vi "Cluster to JSON.vi"(8 "error in":errorcluster, 11 "Mouse Data":T2) -> (0 "error out":errorcluster, 3 "JSON":string)   [LabVIEW 2011]
uses:
  <vilib>/Utility/GetType.llb/Type Enum.ctl
  Mouse Data Cluster.ctl
  <vilib>/vision/Image Controls.llb/IMAQ Image.ctl
  Downloads/JSON.lvlib
  <vilib>/Utility/VariantDataType/VariantType.lvlib
panel:
  out "Array":T1[](array[typedef])
  out "Type Enum":T1=enum."String"
  out "Numeric":i32
  out "Label.Text":string
  out "value":string
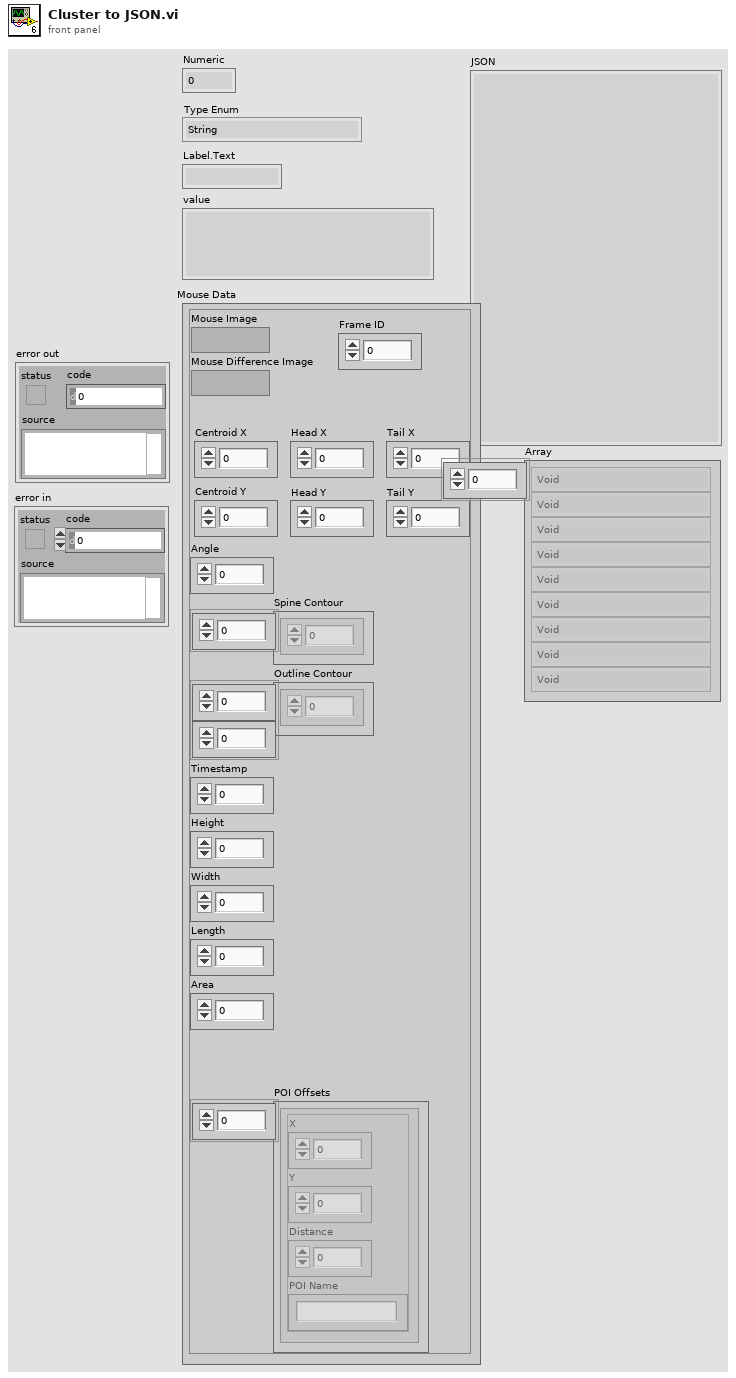
[diagram p1: front panel]
types:
  T1 = typedef "Type Enum.ctl" = enum8{"Void", "I8", "I16", "I32", "I64", "U8", "U16", "U32", "U64", "Single Float", "Double Float", "Extended Float", "Single Complex", "Double Complex", "Extended Complex", "Enum I8 NEVER", "Enum I16 NEVER", "Enum I32 NEVER", "Enum I64 NEVER", "Enum U8", "Enum U16", "Enum U32", "Enum U64", "Single Float With Unit", "Double Float With Unit", "Extended Float With Unit", "Single Complex With Unit", "Double Complex With Unit", "Extended Complex With Unit", "boolU16", "Boolean", "String", "Handle", "Path", "Picture", "C String", "Pascal String", "Tag", "SubString", "Array", "SubArray", "Cluster", "Numeric Cluster", "Variant", "LV Variant", "Measure Data (waveform)", "Refnum", "ExtData", "function", "Typedef", "Poly VI", "bad wire", "LabVIEW Class Instance"}
  T2 = typedef "Mouse Data Cluster.ctl" = cluster{"Mouse Image":T3, "Mouse Difference Image":T3, "Angle":i32, "Spine Contour":i32[], "Outline Contour":i32[][], "Timestamp":dbl, "Height":i32, "Width":i32, "Length":i32, "Area":sgl, "POI Offsets":cluster{"X":i32, "Y":i32, "Distance":i32, "POI Name":string}[], "Frame ID":i16, "Centroid X":i32, "Centroid Y":i32, "Head X":i32, "Head Y":i32, "Tail X":i32, "Tail Y":i32}
  T3 = typedef "IMAQ Image.ctl" = refnum<image>
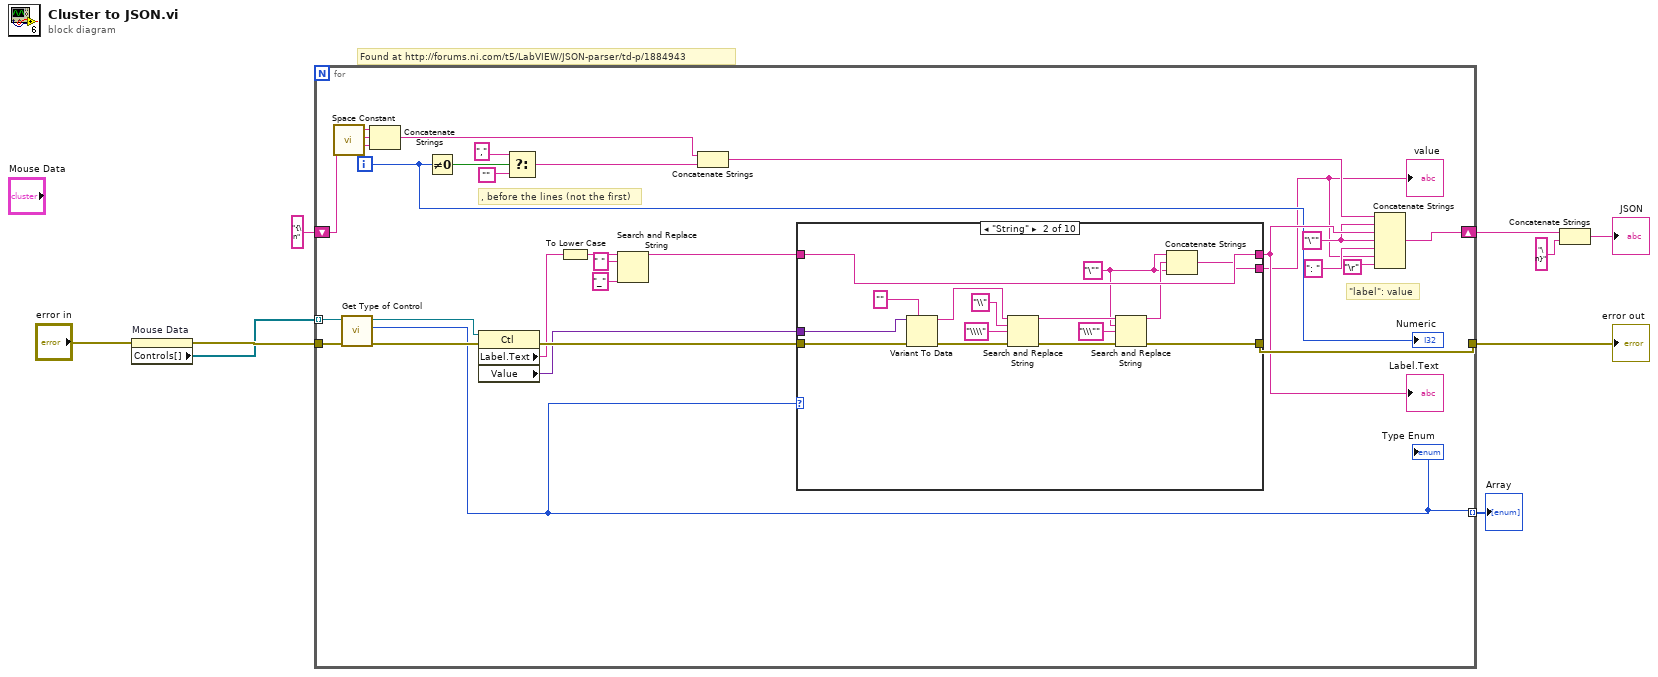
[diagram p0: block diagram]
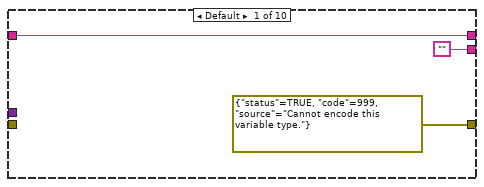
[diagram p2: hidden frame]
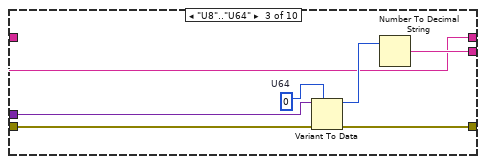
[diagram p3: hidden frame]
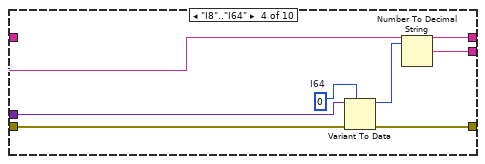
[diagram p4: hidden frame]
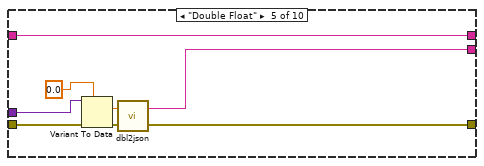
[diagram p5: hidden frame]
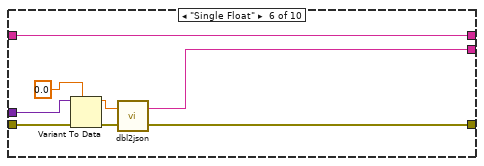
[diagram p6: hidden frame]
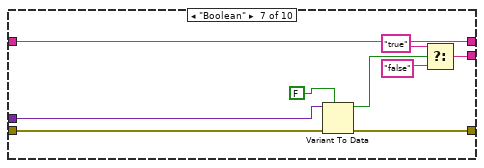
[diagram p7: hidden frame]
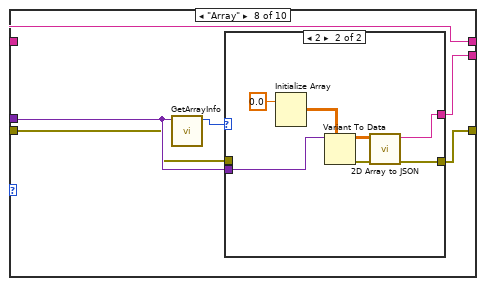
[diagram p8: hidden frame]
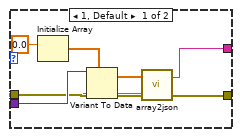
[diagram p9: hidden frame]
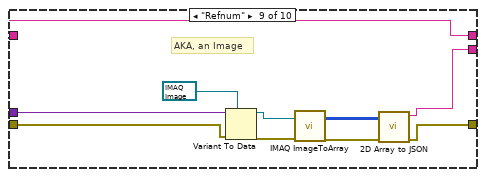
[diagram p10: hidden frame]
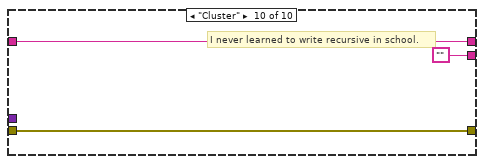
[diagram p11: hidden frame]
diagram:
  # "Found at http://forums.ni.com/t5/LabVIEW/JSON-parser/td-p/1884943"
  n1 = property on="Mouse Data" class="Clust (strict)"(error in="error in") -> (error out=w3:errorcluster, "Controls[]"=w2:refnum<vi>[])  [unwired: 1 in, 1 out]
  n2 = for {
    tunnel: w2 -> [w37] mode=indexing
    tunnel: w3 -> [w36]
    tunnel: [w32] -> w9
    shift-right: [w31] -> w7
    shift-left: "{\n" -> [w21]
    tunnel: [w15] -> w1 mode=indexing
    i -> [w26]
    w28 = "\""
    # ", before the lines (not the first)"
    # "\"label\": value"
    n3 = call <vilib>:"Space Constant.vi"() -> ("String"=w19:string)
    n4 = call <vilib>:"Get Type of Control.vi"("error in (no error)"=w36, "Control Ref In"=w37) -> ("error out"=w34:errorcluster, "Type Enum"=w15:T1, "Control Ref Out"=w35:refnum<vi>)  [unwired: 7 in]
    "Type Enum" <- w15
    n5 = Concatenate Strings(w21, w19, w19) -> (w20:string)
    n6 = Not Equal To 0?(x=w26) -> (x != 0?=w27:bool)
    n7 = property class="Ctl"(reference=w35, error in=w34) -> (error out=w33:errorcluster, "Label.Text"=w14:string, "Value"=w18:variant)  [unwired: 1 out]
    n8 = Select(t=",", s=w27, f="") -> (s? t:f=w25:string)
    n9 = To Lower Case(string=w14) -> (all lower case string=w13:string)
    n10 = Search and Replace String(input string=w13, search string=" ", replace string="_" ("replace string (\"\")")) -> (result string=w10:string)  [unwired: 5 in, 3 out]
    n11 = Concatenate Strings(w20, w25) -> (w22:string)
    n12 = case shown="\"String\"" w15 {
      tunnel: ["" w43 w60 w67 w70 w78 w90 w96 w117 ""] -> w17
      tunnel: [w40 w53 w59 w66 w76 w84 w89 w100 w125 w128] -> w30
      tunnel: w18 -> [_ w54 w58 w65 w74 w82 w87 w98 w123 _]
      tunnel: w10 -> [w40 w53 w59 w66 w76 w84 w89 w100 w125 w128]
      tunnel: w33 -> [_ w52 w57 w64 w75 w83 w88 w97 w122 w126]
      tunnel: [errorcluster {"status"=TRUE, "code"=999, "source"="Cannot encode this variable type."} ("error constant") w45 w56 w63 w71 w79 w86 w95 w116 w126] -> w32
      frame Default {
      }
      frame "String" {
        w41 = "\"" ("search string")
        n13 = Variant To Data(error in=w52, type="", Variant=w54) -> (data=w51:string, error out=w48:errorcluster)
        n14 = Search and Replace String(input string=w51, search string="\\", replace string="\\\\" ("replace string (\"\")"), error in=w48) -> (result string=w47:string, error out=w46:errorcluster)  [unwired: 4 in, 2 out]
        n15 = Search and Replace String(input string=w47, search string=w41, replace string="\\\"" ("replace string (\"\")"), error in=w46) -> (result string=w42:string, error out=w45:errorcluster)  [unwired: 4 in, 2 out]
        n16 = Concatenate Strings(w41, w42, w41) -> (w43:string)
      }
      frame "U8".."U64" {
        w62 = u64 0  # U64
        n17 = Variant To Data(error in=w57, type=w62, Variant=w58) -> (data=w61:u64, error out=w56:errorcluster)
        n18 = Number To Decimal String(number=w61) -> (decimal integer string=w60:string)  [unwired: 1 in]
      }
      frame "I8".."I64" {
        w69 = i64 0  # I64
        n19 = Variant To Data(error in=w64, type=w69, Variant=w65) -> (data=w68:i64, error out=w63:errorcluster)
        n20 = Number To Decimal String(number=w68) -> (decimal integer string=w67:string)  [unwired: 1 in]
      }
      frame "Double Float" {
        n21 = Variant To Data(error in=w75, type=0.0, Variant=w74) -> (data=w73:dbl, error out=w72:errorcluster)
        n22 = call "dbl2json.vi"("error in (no error)"=w72, "Numeric"=w73) -> ("error out"=w71:errorcluster, "JSON"=w70:string)
      }
      frame "Single Float" {
        n23 = Variant To Data(error in=w83, type=0.0, Variant=w82) -> (data=w81:dbl, error out=w80:errorcluster)
        n24 = call "dbl2json.vi"("error in (no error)"=w80, "Numeric"=w81) -> ("error out"=w79:errorcluster, "JSON"=w78:string)
      }
      frame "Boolean" {
        n25 = Variant To Data(error in=w88, type=FALSE, Variant=w87) -> (data=w93:bool, error out=w86:errorcluster)
        n26 = Select(t="true", s=w93, f="false") -> (s? t:f=w90:string)
      }
      frame "Array" {
        n27 = call <vilib>:"GetArrayInfo.vi"("Variant"=w98) -> ("NDims"=w99:i32)  [unwired: 7 in, 3 out]
        n28 = case shown="2" w99 {
          tunnel: w98 -> [w106 w113]
          tunnel: w97 -> [w103 _]
          tunnel: [w102 w111] -> w96
          tunnel: [w101 w109] -> w95
          frame 1, Default {
            n29 = Initialize Array(0.0 ("element")) -> (w108:dbl[])  [unwired: 1 in]
            n30 = Variant To Data(error in=w103, type=w108, Variant=w106) -> (data=w105:dbl[], error out=w104:errorcluster)
            n31 = call "array2json.vi"("error in (no error)"=w104, "Array in"=w105) -> ("error out"=w101:errorcluster, "JSON"=w102:string)
          }
          frame 2 {
            n32 = Initialize Array(0.0 ("element")) -> (w115:dbl[][])  [unwired: 2 in]
            n33 = Variant To Data(type=w115, Variant=w113) -> (data=w112:dbl[][], error out=w110:errorcluster)  [unwired: 1 in]
            n34 = call "2D Array to JSON.vi"("error in"=w110, "Array"=w112) -> ("error out"=w109:errorcluster, "String"=w111:string)  [unwired: 8 in]
          }
        }
      }
      frame "Refnum" {
        # "AKA, an Image"
        n35 = Variant To Data(error in=w122, type=T3 refnum ("Image"), Variant=w123) -> (data=w121:T3, error out=w120:errorcluster)
        n36 = call "IMAQ ImageToArray"("error in (no error)"=w120, "Image"=w121) -> ("error out"=w118:errorcluster, "Image Pixels (I16)"=w119:i16[][])  [unwired: 2 in, 3 out]
        n37 = call "2D Array to JSON.vi"("error in"=w118, "Array"=w119) -> ("error out"=w116:errorcluster, "String"=w117:string)  [unwired: 8 in]
      }
      frame "Cluster" {
        # "I never learned to write recursive in school."
      }
    }
    "Label.Text" <- w30
    "value" <- w17
    n38 = Concatenate Strings(w22, w28, w30, w28, ": ", w17, "\r") -> (w31:string)
    "Numeric" <- w26
  }
  "error out" <- w9
  "Array" <- w1
  n39 = Concatenate Strings(w7, "\n}") -> (→"JSON":string)
